vi "Create DebugTerminal.vi"(7 "PacketFormatter":refnum<class "PacketFormatter.lvclass">, 8 "error in (no error)":errorcluster, 11 "DebuggingTerminal in":refnum<class "DebuggingTerminal.lvclass">) -> (0 "error out":errorcluster, 3 "DebuggingTerminal out":refnum<class "DebuggingTerminal.lvclass">)   [LabVIEW 2013, in "MQTT Base.lvlib" / "DebuggingTerminal.lvclass"]
uses:
  DebuggingTerminal.lvclass
  PacketFormatter/PacketFormatter.lvclass
  DebuggingTerminal.lvclass/DebuggingTerminal.ctl
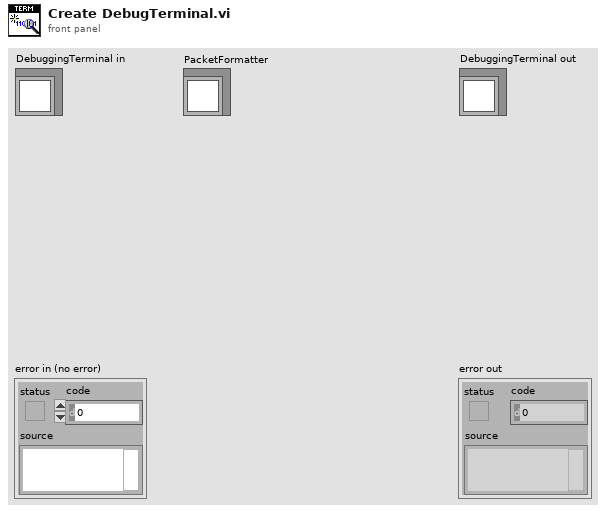
[diagram p1: front panel]
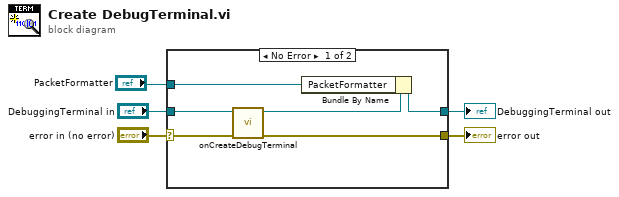
[diagram p0: block diagram]
diagram:
  n1 = case shown="No Error" "error in (no error)" {
    selector: "error in (no error)" -> [w10 w13]
    tunnel: [w9 w13] -> w4
    tunnel: [w6 w12] -> w2
    tunnel: "DebuggingTerminal in" -> [w11 w12]
    tunnel: "PacketFormatter" -> [w8 _]
    frame No Error {
      n2 = call-dynamic "onCreateDebugTerminal.vi"("error in (no error)"=w10, "DebuggingTerminal in"=w11) -> ("error out"=w9:errorcluster, "DebuggingTerminal out"=w7:refnum<class "DebuggingTerminal.lvclass">)  [unwired: 8 in]
      n3 = Bundle By Name(cluster=w7, "PacketFormatter"=w8) -> (w6:refnum<class "DebuggingTerminal.lvclass">)
    }
    frame Error {
    }
  }
  "error out" <- w4
  "DebuggingTerminal out" <- w2
